vi "Teleop.vi"   [LabVIEW 2013]
doc: "This VI is called for each TeleOp packet received from the DS where the robot is not disabled. It is often used to read from the joysticks and update I/O or to update setpoints for timed control loops. It should complete and return within 20 milliseconds or it may miss DS packets."
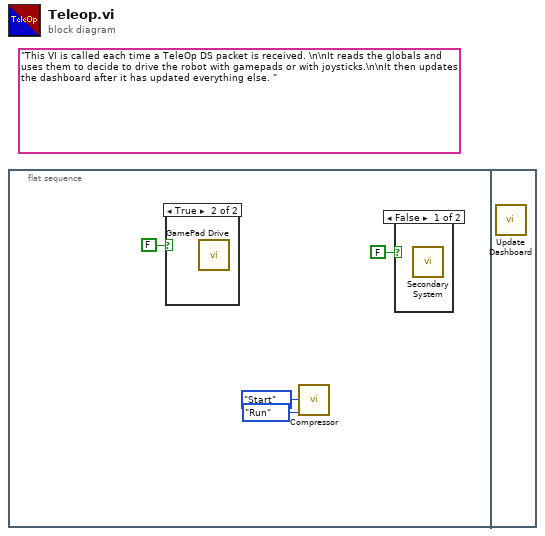
[diagram p0: block diagram]
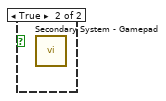
[diagram p2: hidden frame]
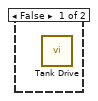
[diagram p3: hidden frame]
diagram:
  (unwired) "This VI is called each time a TeleOp DS packet is received. \n\nIt reads the globals and uses them to decide to drive the robot with gamepads or with joysticks.\n\nIt then updates the dashboard after it has updated everything else. "
  n1 = flat-sequence {
    frame #0 {
      n2 = case shown="True" FALSE {
        frame False {
          n3 = call "Tank Drive.vi"() -> ()  [unwired: 12 out]
        }
        frame True {
          n4 = call "GamePad Drive.vi"() -> ()  [unwired: 12 out]
        }
      }
      n5 = call "Compressor.vi"("Mode"=enum16{"Init", "Run", "End"}."Run", "Compressor State"=enum32{"Start", "Stop"}."Start") -> ()  [unwired: 10 in]
      n6 = case shown="False" FALSE {
        frame False {
          n7 = call "Secondary System.vi"() -> ()  [unwired: 12 out]
        }
        frame True {
          n8 = call "Secondary System - Gamepad.vi"() -> ()  [unwired: 1 in, 11 out]
        }
      }
    }
    frame #1 {
      n9 = call "Update Dashboard.vi"() -> ()  [unwired: 12 out]
    }
  }
